vi "ReadDestinations.vi"(8 "Error In":errorcluster, 11 "object in":refnum<class "Module.lvclass">) -> (0 "Error Out":errorcluster, 2 "Destinations":string[](array[string]), 3 "object out":refnum<class "Module.lvclass">)   [LabVIEW 2021, in "Module.lvclass"]
uses:
  Module.lvclass
  Module.lvclass/Module.ctl
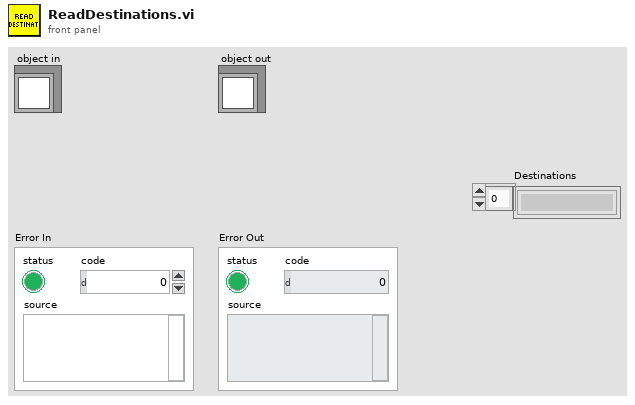
[diagram p1: front panel]
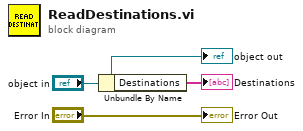
[diagram p0: block diagram]
diagram:
  n1 = Unbundle By Name("object in") -> ("Destinations"=→"Destinations":string[])
  "Error Out" <- "Error In"
  "object out" <- "object in"
